vi "13HB_EnFlo_Specific.vi"(8 "Data rate (Hz)":dbl=50.0, 9 "N samples":i32=500, 11 "COM Port":refnum<visa-resource-name>) -> (0 "I/O error":errorcluster, 1 "All chksums ok":bool, 2 "Avg. data rate (Hz)":dbl format="%#_3g", 3 "Data":sgl[][](array[numeric]))   [LabVIEW 2018]
uses:
  5HC/ctls/Cmds.ctl
panel:
  out "Chksum":bool[](array[boolean])
  out "Loop period (ms)":dbl format="%#_3g"
  out "T0 (°C)":sgl[](array[numeric]) format="%#.2g"
  out "Vb":sgl[][](graph)
  in  "Stop Button":bool
  # "Data array output format:\n\nVb1\nT1\n.\n.\nVb13\nT13\nP_atm1\nRH1\n{ax1, ay1, az1\n{wx,1 wy1, wz1}"
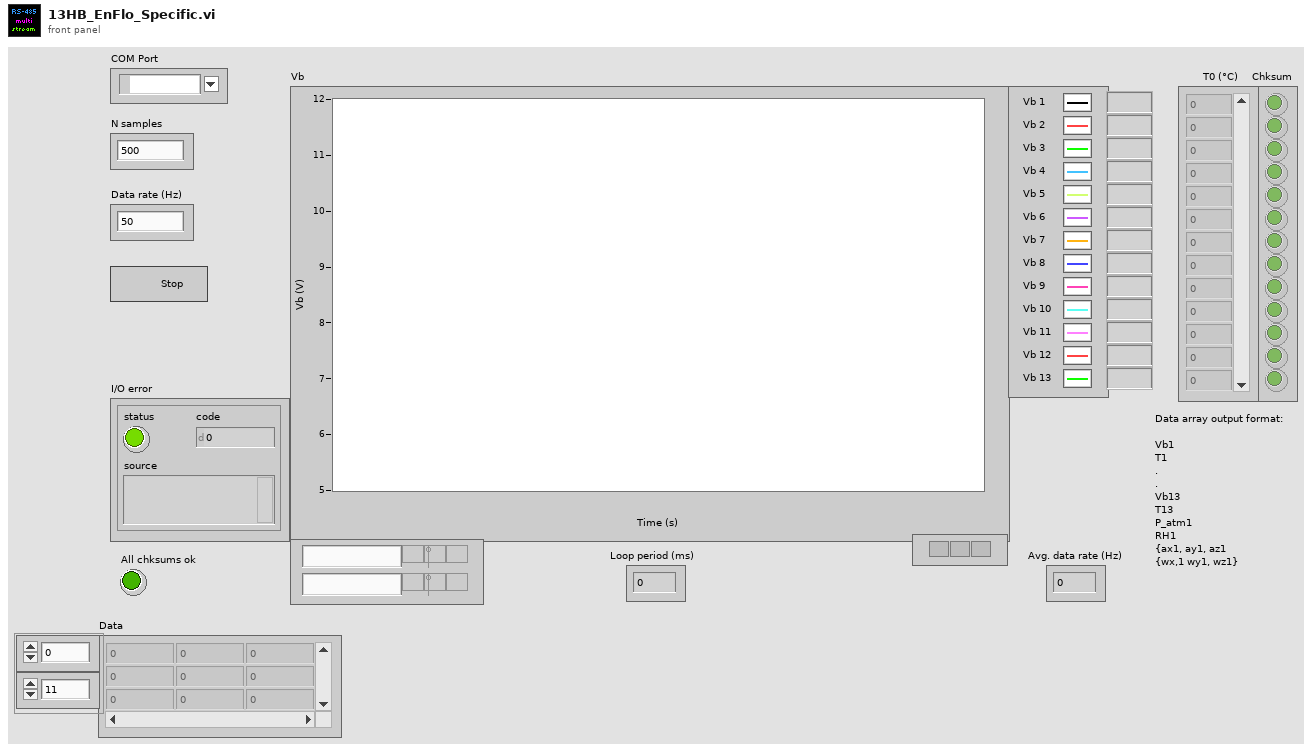
[diagram p1: front panel]
types:
  T1 = typedef "Cmds.ctl" = u8
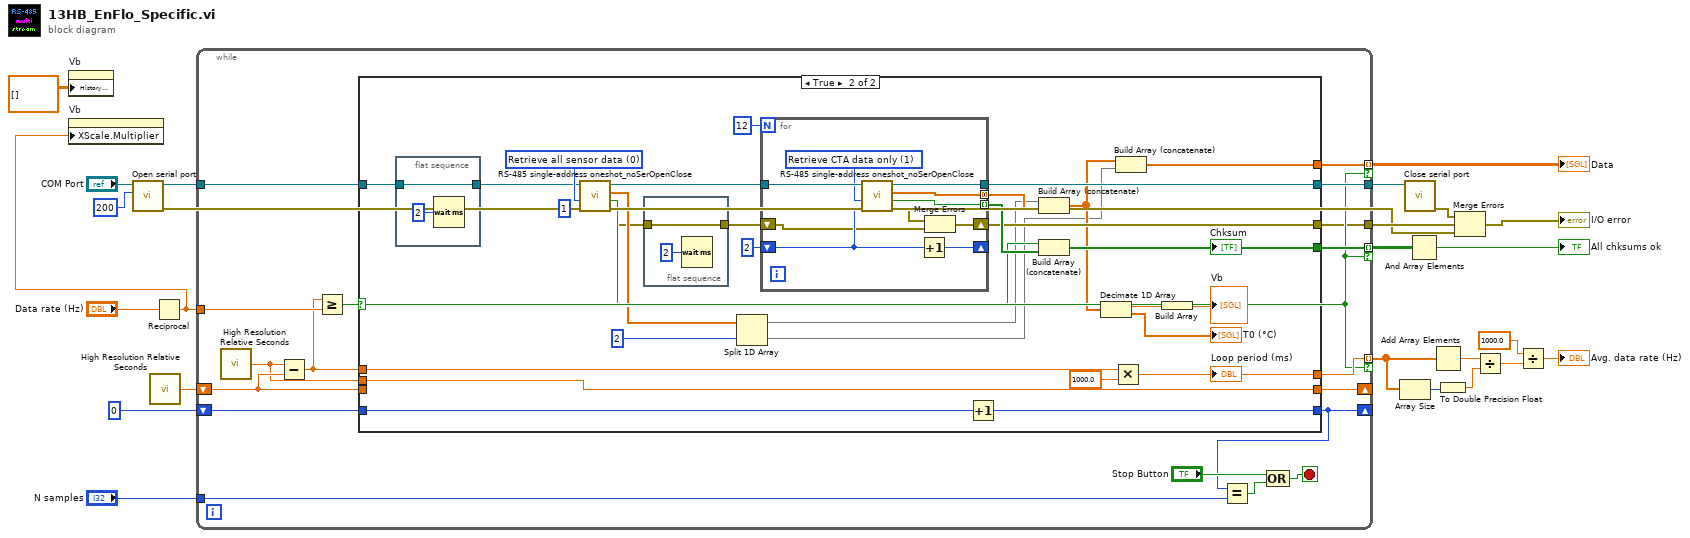
[diagram p0: block diagram]
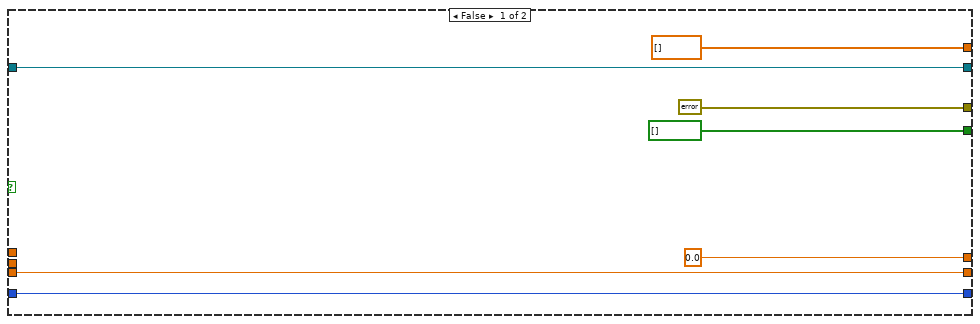
[diagram p2: hidden frame]
diagram:
  n1 = property on="Vb" class="WFChart (strict)"("History Data"=sgl[][] []) -> ()  [unwired: 2 in, 2 out]
  n2 = call "Open serial port.vi"("timeout (ms)"=u32 200, "VISA resource name"="COM Port") -> ("Error out"=w11:errorcluster, "VISA resource name out"=w1:refnum<visa-resource-name>)  [unwired: 8 in]
  n3 = call <vilib>:"High Resolution Relative Seconds.vi"() -> ("relative seconds"=w24:dbl)
  n4 = Reciprocal(x="Data rate (Hz)") -> (1/x=w2:dbl)
  n5 = property on="Vb" class="WFChart (strict)"("XScale.Multiplier"=w2) -> ()  [unwired: 2 in, 2 out]
  n6 = while {
    tunnel: w2 -> [w39]
    shift-right: [w40] -> _
    shift-left: w24 -> [w42]
    tunnel: [w37] -> w19
    tunnel: "N samples" -> [w28]
    tunnel: [w33] -> w17 mode=indexing if=w30
    tunnel: [w32] -> w16 mode=indexing if=w30
    tunnel: [w26] -> w12
    tunnel: [w31] -> w8 mode=indexing if=w30
    shift-right: [w27] -> _
    shift-left: 0 ("N samples") -> [w29]
    tunnel: w1 -> [w25]
    stop <- w35 stop-if-true
    n7 = call <vilib>:"High Resolution Relative Seconds.vi"() -> ("relative seconds"=w41:dbl)
    n8 = Subtract(x=w41, y=w42) -> (x-y=w38:dbl)
    n9 = Greater Or Equal?(x=w38, y=w39) -> (x >= y?=w30:bool)
    n10 = case shown="True" w30 {
      tunnel: [errorcluster {"status"=FALSE, "code"=0, "source"=""} ("I/O error") w67] -> w26
      tunnel: w38 -> [_ w78]
      tunnel: w42 -> [w49 _]
      tunnel: w41 -> [_ w79]
      tunnel: [w49 w79] -> w40
      tunnel: [w43 w71] -> w37
      tunnel: [sgl[] [] w60] -> w33
      tunnel: [bool[] [] w66] -> w32
      tunnel: [0.0 w56] -> w31
      tunnel: [w44 w55] -> w27
      tunnel: w29 -> [w44 w54]
      tunnel: w25 -> [w43 w51]
      frame False {
      }
      frame True {
        w76 = T1 0 items=["Retrieve all sensor data", "Retrieve CTA data only", "USB streaming enable", "USB streaming disable", "Retrieve EEPROM table", "Set address byte", "Get address byte", "Run self-test"] ("Command")
        n11 = flat-sequence {
          tunnel: [w80] -> w50
          tunnel: w51 -> [w80]
          frame #0 {
            n12 = Wait (ms)(milliseconds to wait=u32 2) -> ()  [unwired: 1 out]
          }
        }
        n13 = call "RS-485 single-address oneshot_noSerOpenClose.vi"("Address"=u8 1, "Command"=w76, "COM Port"=w50) -> ("I/O error"=w52:errorcluster, "Checksum ok"=w69:bool, "Data"=w65:sgl[], "COM Port out"=w74:refnum<visa-resource-name>)  [unwired: 1 in]
        n14 = flat-sequence {
          tunnel: [w82] -> w53
          tunnel: w52 -> [w82]
          frame #0 {
            n15 = Wait (ms)(milliseconds to wait=u32 2) -> ()  [unwired: 1 out]
          }
        }
        n16 = Split 1D Array(array=w65, index=2) -> (first subarray=w63:sgl[], second subarray=w61:sgl[])
        n17 = for {
          N: 12 -> [_]
          tunnel: w74 -> [w93]
          shift-right: [w91] -> _
          shift-left: u8 2 ("Address") -> [w90]
          shift-right: [w88] -> w67
          shift-left: w53 -> [w87]
          tunnel: [w86] -> w70 mode=indexing
          tunnel: [w85] -> w71
          tunnel: [w84] -> w68 mode=concatenating
          w92 = T1 1 items=["Retrieve all sensor data", "Retrieve CTA data only", "USB streaming enable", "USB streaming disable", "Retrieve EEPROM table", "Set address byte", "Get address byte", "Run self-test"] ("Command")
          n18 = call "RS-485 single-address oneshot_noSerOpenClose.vi"("Address"=w90, "Command"=w92, "COM Port"=w93) -> ("I/O error"=w89:errorcluster, "Checksum ok"=w86:bool, "Data"=w84:sgl[], "COM Port out"=w85:refnum<visa-resource-name>)  [unwired: 1 in]
          n19 = Increment(x=w90) -> (x+1=w91:u8)
          n20 = Merge Errors(w89, w87) -> (w88:errorcluster)
        }
        n21 = Increment(x=w54) -> (x+1=w55:i32)
        n22 = Build Array (concatenate)(w63, w68) -> (w62:sgl[])
        n23 = Build Array (concatenate)(w69, w70) -> (w66:bool[])
        "Chksum" <- w66
        n24 = Decimate 1D Array(w62) -> (w59:sgl[], →"T0 (°C)":sgl[])
        n25 = Multiply(x=w78, y=1000.0) -> (x*y=w56:dbl)
        "Loop period (ms)" <- w56
        n26 = Build Array (concatenate)(w62, w61) -> (w60:sgl[])
        n27 = Build Array(w59) -> (→"Vb":sgl[][])
      }
    }
    n28 = Equal?(x=w27, y=w28) -> (x = y?=w34:bool)
    n29 = Compound Arithmetic op=OR("Stop Button", w34) -> (w35:bool)
  }
  "Data" <- w17
  n30 = Array Size(array=w8) -> (size(s)=w7:i32)
  n31 = call "Close serial port.vi"("VISA resource name"=w19) -> ("Error out"=w14:errorcluster)  [unwired: 10 in]
  n32 = And Array Elements(Boolean array=w16) -> (logical AND=→"All chksums ok":bool)
  n33 = Add Array Elements(numeric array=w8) -> (sum=w10:dbl)
  n34 = To Double Precision Float(number=w7) -> (double precision float=w9:dbl)
  n35 = Merge Errors(w14, w12, w11) -> (→"I/O error":errorcluster)
  n36 = Divide(x=w10, y=w9) -> (x/y=w5:dbl)
  n37 = Divide(x=1000.0, y=w5) -> (x/y=→"Avg. data rate (Hz)":dbl)
